vi "data array.vi"() -> (2 "Array":dbl[][](array[numeric]))   [LabVIEW 2021]
uses:
  <vilib>/numeric/Random Number (Range) DBL.vi
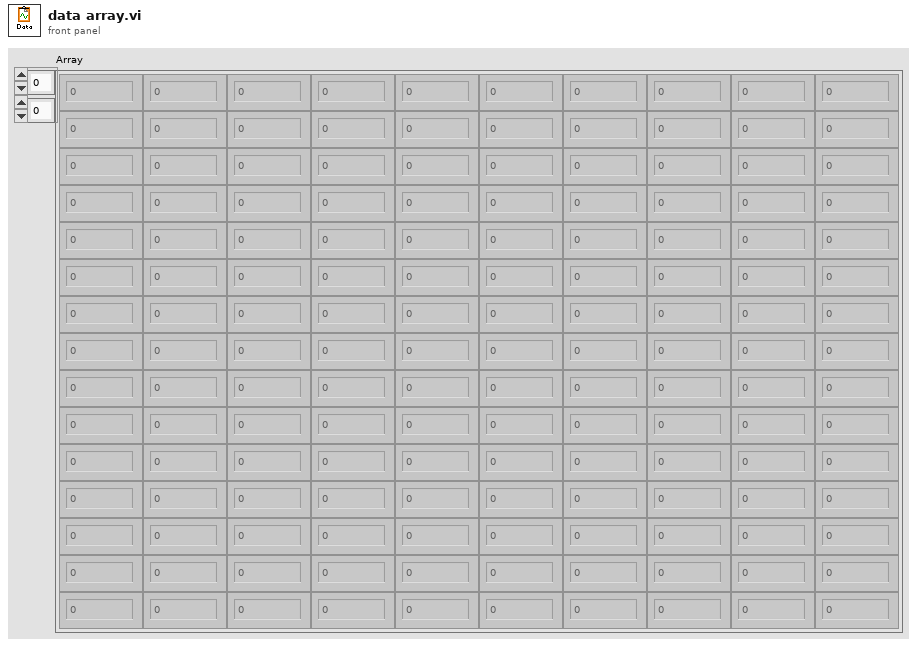
[diagram p1: front panel]
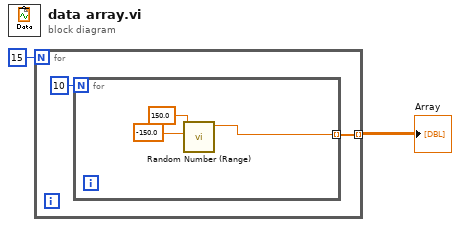
[diagram p0: block diagram]
diagram:
  n1 = for {
    N: 15 -> [_]
    tunnel: [w3] -> w1 mode=indexing
    n2 = for {
      N: 10 -> [_]
      tunnel: [w5] -> w3 mode=indexing
      n3 = call-poly <vilib>:"Random Number (Range).vi"("lower bound (0)"=-150.0, "upper bound (100)"=150.0) -> ("number"=w5:dbl)  [unwired: 9 in]
    }
  }
  "Array" <- w1
